vi "BRig_dataExp_Cue2Switch_First.vi"() -> (2 "output_Cue2Switch_First":i32)   [LabVIEW 2014]
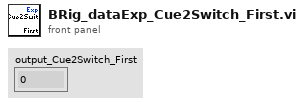
[diagram p1: front panel]
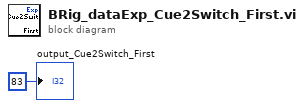
[diagram p0: block diagram]
diagram:
  "output_Cue2Switch_First" <- 83 ("output_iBlock")
